vi "AlliGator Get Tabulated Results Header (Average Lifetimes).vi"(8 "Error In":errorcluster) -> (0 "Error Out":errorcluster, 3 "Tabulated Results Header":string)   [LabVIEW 2021, in "AlliGator Decay Processing.lvlib"]
doc: "Builds string to output results of average lifetime calculation."
uses:
  AlliGator Decay Processing.lvlib
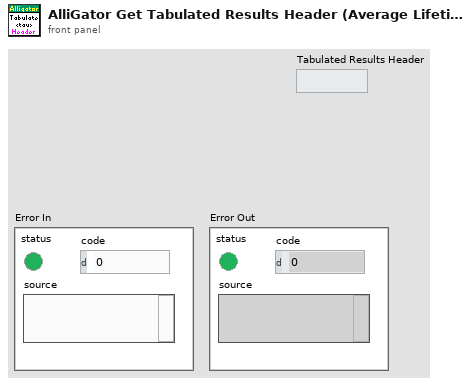
[diagram p1: front panel]
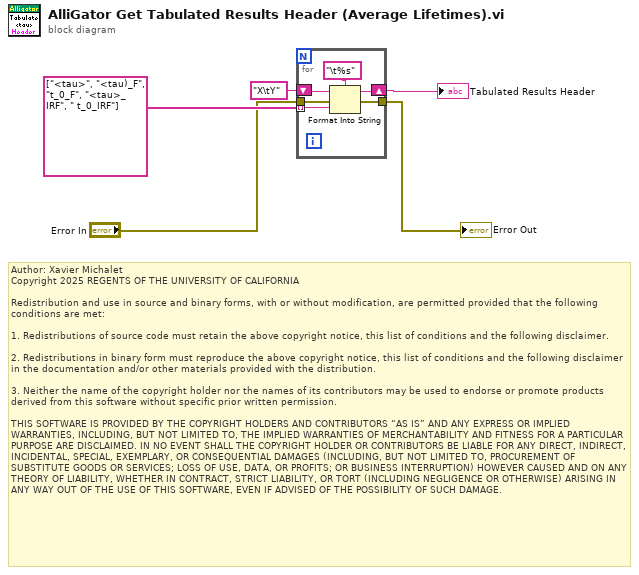
[diagram p0: block diagram]
diagram:
  # "Author: Xavier Michalet\nCopyright 2025 REGENTS OF THE UNIVERSITY OF CALIFORNIA\n\nRedistribution and use in source and binary forms, with or without modification, are permitted provided that the following conditions are met:\n\n1. Redistributions of source code must retain the above copyright notice, this list of conditions and the following disclaimer.\n\n2. Redistributions in binary form must reproduce the above copyright notice, this list of conditions and the following disclaimer in the documentation and/or other materials provided with the distribution.\n\n3. Neither the name of the copyright holder nor the names of its contributors may be used to endorse or promote products derived from this software without specific prior written permission.\n\nTHIS SOFTWARE IS PROVIDED BY THE COPYRIGHT HOLDERS AND CONTRIBUTORS “AS IS” AND ANY EXPRESS OR IMPLIED WARRANTIES, INCLUDING, BUT NOT LIMITED TO, THE IMPLIED WARRANTIES OF MERCHANTABILITY AND FITNESS FOR A PARTICULAR PURPOSE ARE DISCLAIMED. IN NO EVENT SHALL THE COPYRIGHT HOLDER OR CONTRIBUTORS BE LIABLE FOR ANY DIRECT, INDIRECT, INCIDENTAL, SPECIAL, EXEMPLARY, OR CONSEQUENTIAL DAMAGES (INCLUDING, BUT NOT LIMITED TO, PROCUREMENT OF SUBSTITUTE GOODS OR SERVICES; LOSS OF USE, DATA, OR PROFITS; OR BUSINESS INTERRUPTION) HOWEVER CAUSED AND ON ANY THEORY OF LIABILITY, WHETHER IN CONTRACT, STRICT LIABILITY, OR TORT (INCLUDING NEGLIGENCE OR OTHERWISE) ARISING IN ANY WAY OUT OF THE USE OF THIS SOFTWARE, EVEN IF ADVISED OF THE POSSIBILITY OF SUCH DAMAGE."
  n1 = for {
    tunnel: string[] ["<tau>", "<tau)_F", "t_0_F", "<tau>_IRF", " t_0_IRF"] ("initial string") -> [w11] mode=indexing
    shift-right: [w8] -> w5
    shift-left: "X\tY" -> [w9]
    tunnel: "Error In" -> [w7]
    tunnel: [w6] -> w1
    n2 = Format Into String(format string="\t%s", initial string=w9, error in=w7, w11) -> (resulting string=w8:string, error out=w6:errorcluster)
  }
  "Tabulated Results Header" <- w5
  "Error Out" <- w1
